vi "setConfiguration.vi"(8 "error in (no error)":errorcluster, 10 "Configuration":variant, 11 "Instrument in":refnum<class "Instrument.lvclass">) -> (0 "error out":errorcluster, 3 "Instrument out":refnum<class "Instrument.lvclass">)   [LabVIEW 2019, in "Instrument.lvlib" / "Instrument.lvclass"]
doc: "Set \"setConfiguration\" to remote Instrument process."
uses:
  Instrument.lvclass
  Typedefs/Instrument.ProtectedCommands--Enum.ctl
  API/Instrument.sendMessageToProcess (variant).vi
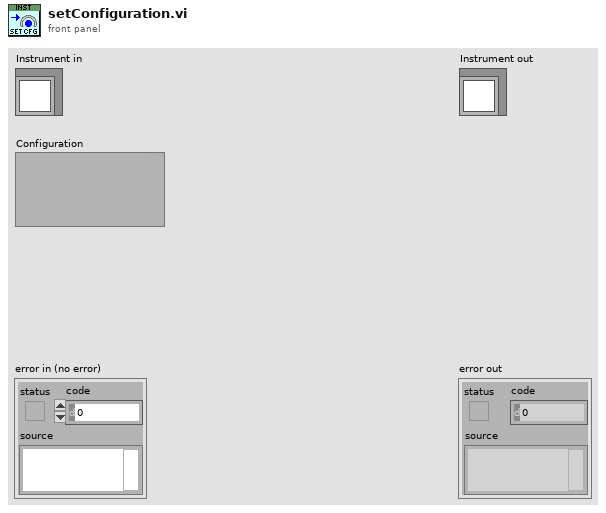
[diagram p1: front panel]
types:
  T1 = typedef "Instrument.lvlib/Instrument.lvclass/Instrument.ProtectedCommands--Enum.ctl" = enum16{"setConfiguration", "setIDN", "setAll", "setAllData"}
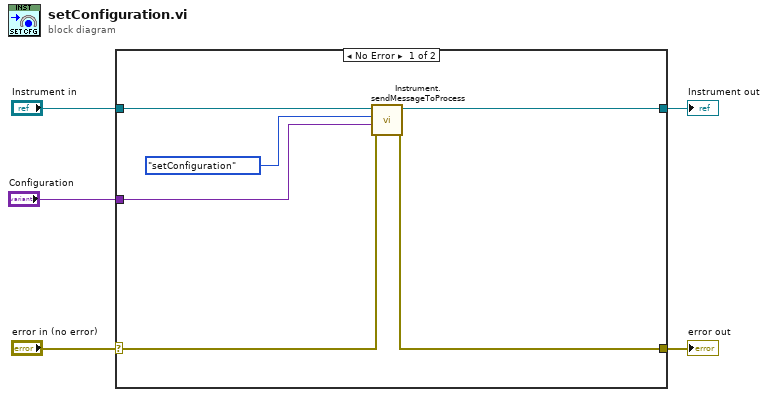
[diagram p0: block diagram]
diagram:
  n1 = case shown="No Error" "error in (no error)" {
    selector: "error in (no error)" -> [w9 w13]
    tunnel: [w7 w13] -> w4
    tunnel: [w8 w12] -> w2
    tunnel: "Instrument in" -> [w6 w12]
    tunnel: "Configuration" -> [w10 _]
    frame No Error {
      n2 = call-poly "Instrument.sendMessageToProcess.vi"("error in (no error)"=w9, "Data"=w10, "Command"=Instrument.ProtectedCommands--Enum."setConfiguration" ("PrivateCommands"), "Instrument"=w6) -> ("error out"=w7:errorcluster, "Instrument out"=w8:refnum<class "Instrument.lvclass">)  [unwired: 6 in]
    }
    frame Error {
    }
  }
  "error out" <- w4
  "Instrument out" <- w2
